vi "configuration UI.vi"() -> ()   [LabVIEW 2013, in "alarms module editor node.lvclass"]
uses:
  alarms module editor node.lvclass
  <vilib>/NI/Module Execution Interface/Engine Configuration/engine configuration.lvclass
  <vilib>/NI/Tag Bus Data Framework/Configuration Editor/Classes/Module editor node/module editor node.lvclass
  <vilib>/NI/Tag Bus Data Framework/Configuration Editor/Classes/Engine Parent/Engine Parent Editor Node.lvclass
  <vilib>/NI/Configuration Framework/serializable configuration/NISE_CEF_serializable configuration.lvclass
  module/configuration/alarms module configuration.lvclass
  <vilib>/NI/Tools/Keyed Array/KeyedArray.ctl
  <vilib>/NI/Tools/Keyed Array/Tools_KeyedArray.lvlib
  <vilib>/NI/AMC/Message.ctl
  <vilib>/NI/AMC/AMC.lvlib
  <vilib>/NI/AMC/Message Queue.ctl
  <vilib>/NI/Configuration Framework/Node/NISE_CEF_Node.lvclass
  <vilib>/NI/Configuration Framework/Node/NodeRef.ctl
  <vilib>/NI/Configuration Framework/Controls/EventCluster.ctl
  <vilib>/NI/Configuration Framework/NISE_CEF_TreeControl.lvlib
  <vilib>/NI/Configuration Framework/Node/UserEventRef.ctl
  <vilib>/NI/Configuration Framework/Node/StopEvent.ctl
  <vilib>/NI/Configuration Framework/Node/RefreshUIEvent.ctl
  <vilib>/NI/Configuration Framework/Node/CacheState.ctl
  <vilib>/NI/Configuration Framework/Node/NodeChangeEvent.ctl
panel:
  in  "node change":T1
  in  "cache state":T2
  in  "refresh UI":T3
  in  "stop event":T4
  in  "Tab Control":enum32{"Alarm Configuration", "Alarm Table"}(tab)
  in  "Alarms":i32(listbox)
  in  "Remove alarm":bool
  in  "Add alarm":bool
  in  "Full Alarms Table":i32(listbox)
  in  "user event":T5
  in  "main queue":T6
  in  "node ref":T7
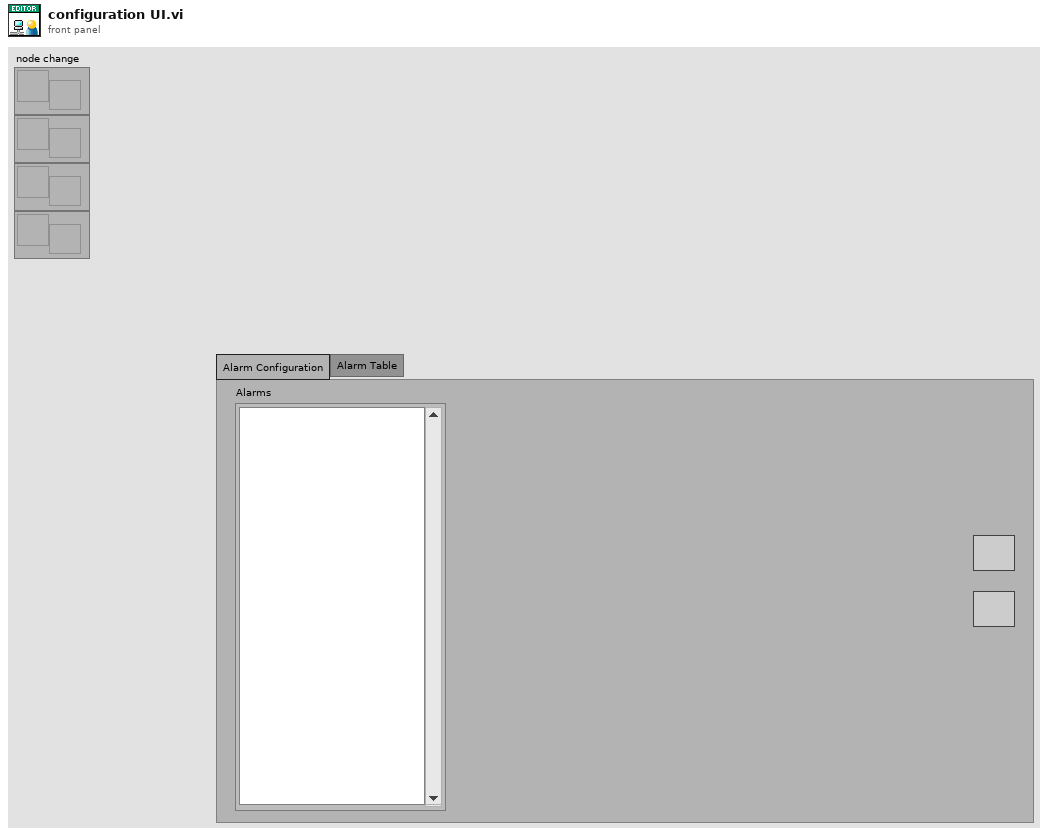
[diagram p1: front panel]
types:
  T1 = typedef "NISE_CEF_Node.lvclass/NodeChangeEvent.ctl" = refnum<user-event>
  T2 = typedef "NISE_CEF_Node.lvclass/CacheState.ctl" = refnum<user-event>
  T3 = typedef "NISE_CEF_Node.lvclass/RefreshUIEvent.ctl" = refnum<user-event>
  T4 = typedef "NISE_CEF_Node.lvclass/StopEvent.ctl" = refnum<user-event>
  T5 = typedef "NISE_CEF_Node.lvclass/UserEventRef.ctl" = refnum<user-event>
  T6 = typedef "AMC.lvlib/Message Queue.ctl" = refnum<queue>
  T7 = typedef "NISE_CEF_Node.lvclass/NodeRef.ctl" = refnum<data-value>
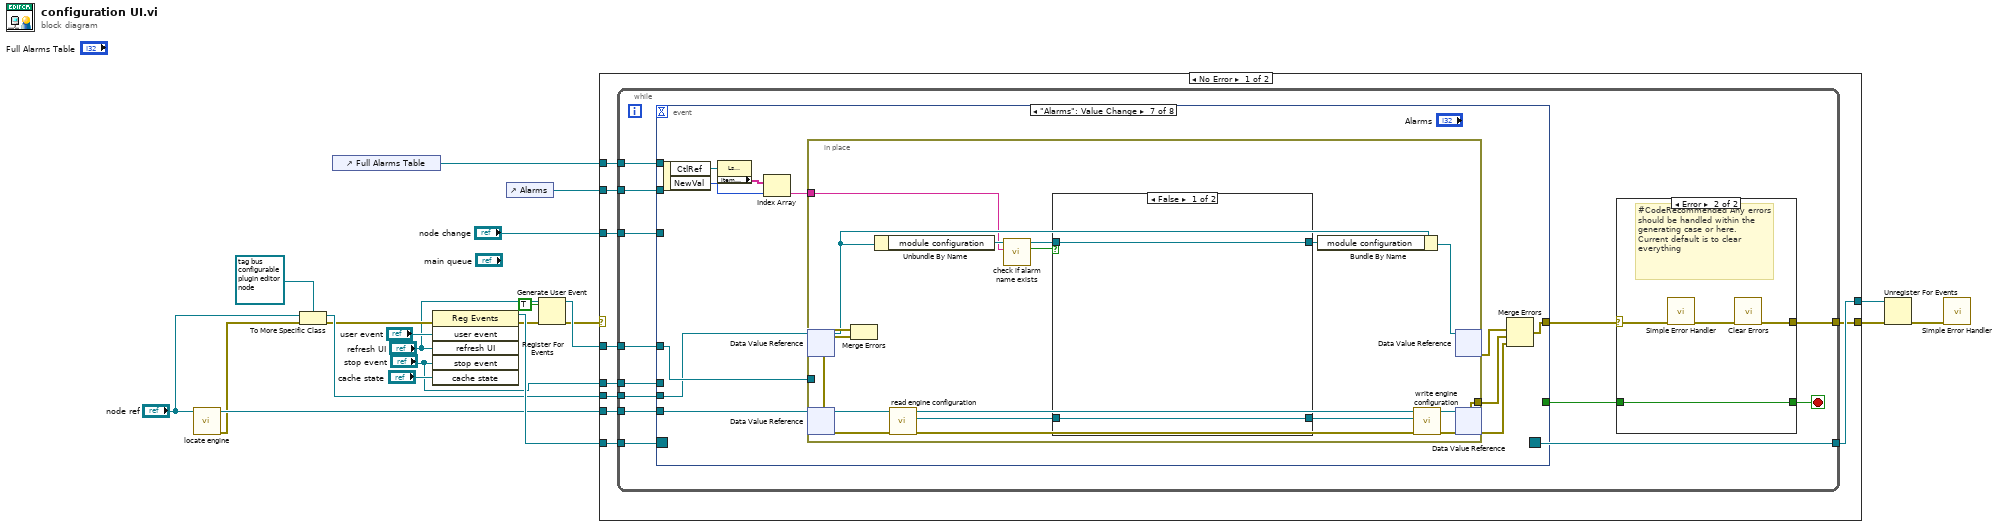
[diagram p0: block diagram]
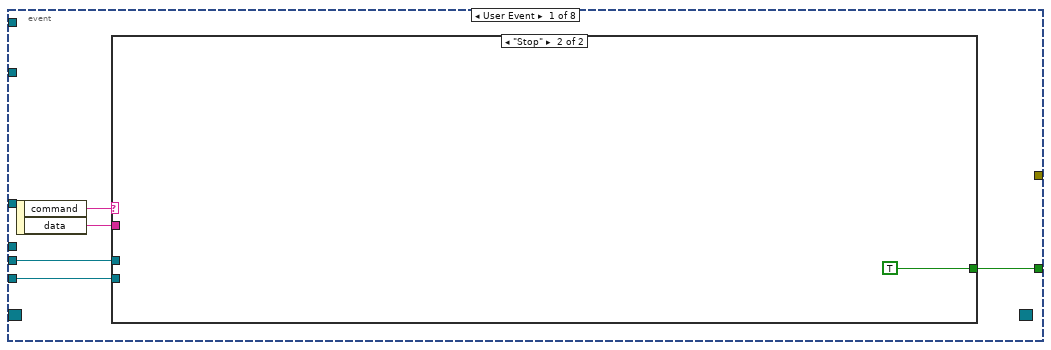
[diagram p3: hidden frame]
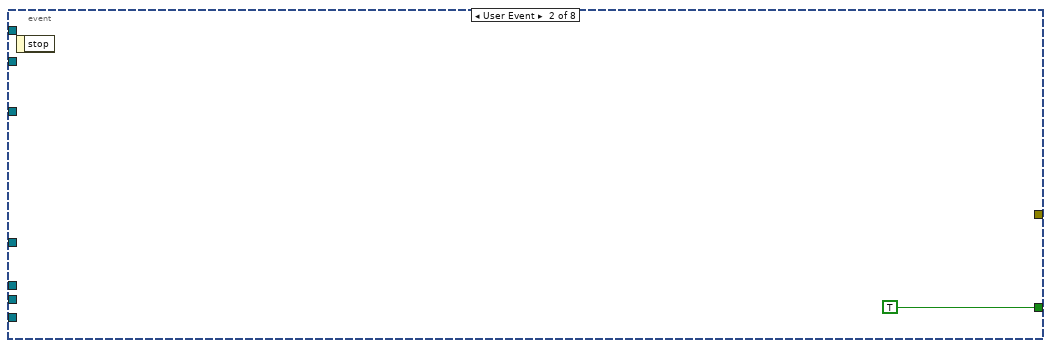
[diagram p5: hidden frame]
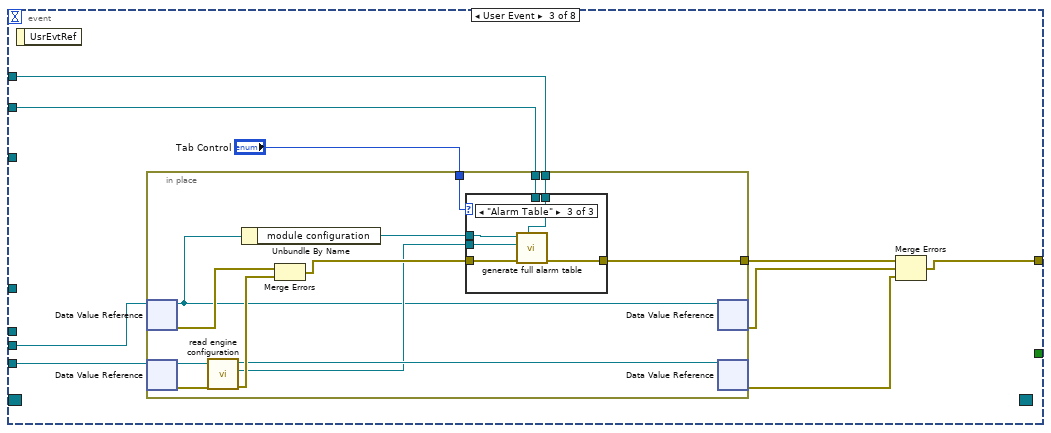
[diagram p6: hidden frame]
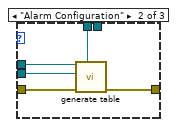
[diagram p8: hidden frame]
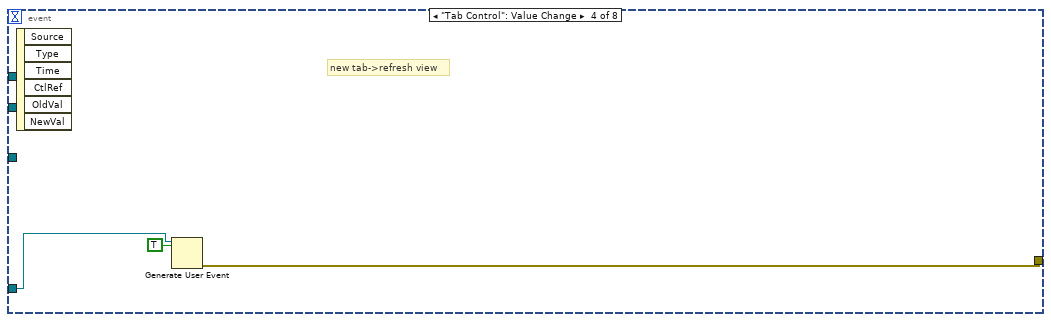
[diagram p9: hidden frame]
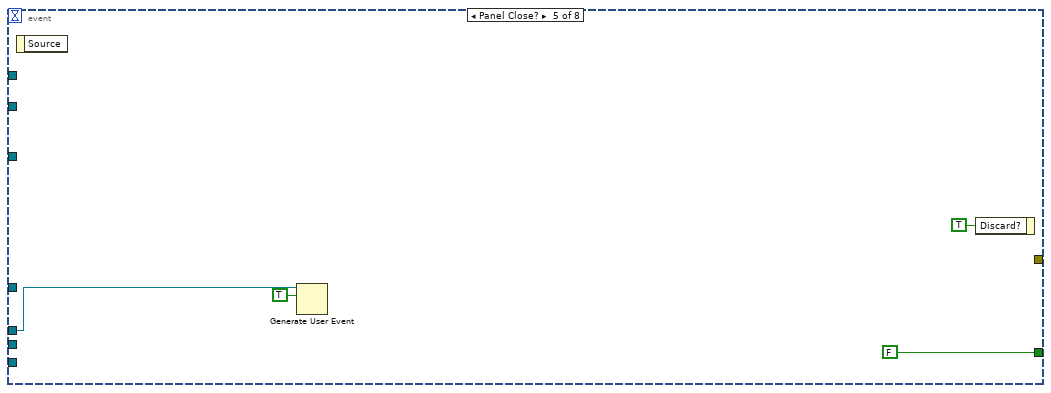
[diagram p10: hidden frame]
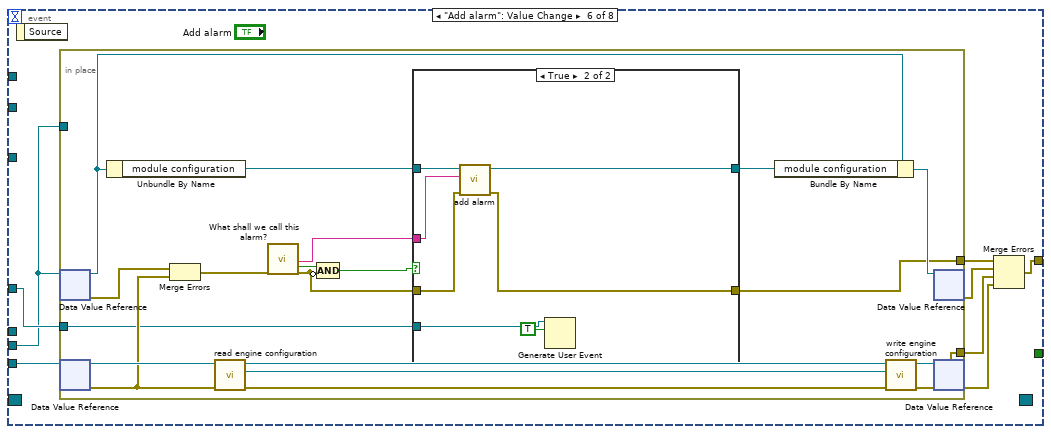
[diagram p11: hidden frame]
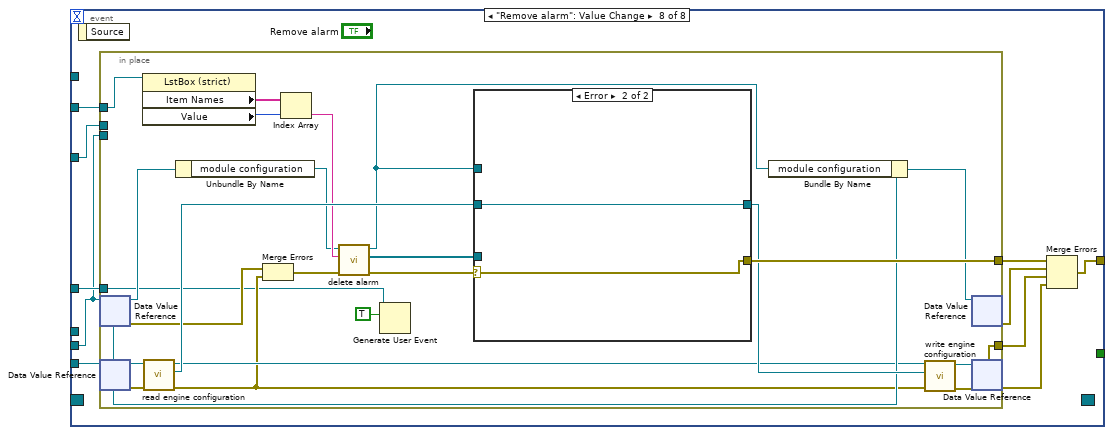
[diagram p14: hidden frame]
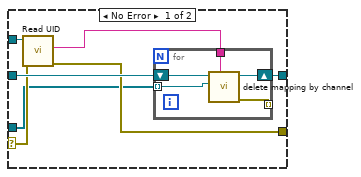
[diagram p15: hidden frame]
diagram:
  n1 = call <vilib>:"locate engine.vi"("component"="node ref") -> ("error out"=w10:errorcluster, "engine"=w16:refnum<data-value>)  [unwired: 9 in]
  n2 = To More Specific Class(target class=refnum<data-value> refnum ("data value reference"), reference="node ref", error in=w10) -> (specific class reference=w13:refnum<data-value>, error out=w12:errorcluster)
  n3 = control-ref of="Full Alarms Table"() -> (w1:refnum<vi>)
  n4 = register-events(error in=w12, "user event", "refresh UI", "stop event", "cache state") -> (reference out=w21:refnum<event-registration>, error out=w17:errorcluster)  [unwired: 1 in]
  n5 = control-ref of="Alarms"() -> (w2:refnum<vi>)
  n6 = Generate User Event(user event="refresh UI", event data cluster=TRUE ("event data"), error in=w17) -> (user event out=w9:T3, error out=w4:errorcluster)  [unwired: 1 in]
  n7 = case shown="No Error" w4 {
    selector: w4 -> [_ w211]
    tunnel: w21 -> [w31 w210]
    tunnel: [w30 w210] -> w20
    tunnel: [w29 w211] -> w19
    tunnel: w16 -> [w28 _]
    tunnel: w13 -> [w27 _]
    tunnel: w9 -> [w26 _]
    tunnel: "node change" -> [w25 _]
    tunnel: "stop event" -> [w24 _]
    tunnel: w2 -> [w23 _]
    tunnel: w1 -> [w22 _]
    frame No Error {
      n8 = while {
        tunnel: w31 -> [w44]
        tunnel: [w43] -> w30
        tunnel: w27 -> [w39]
        tunnel: w28 -> [w38]
        tunnel: w26 -> [w37]
        tunnel: w25 -> [w35]
        tunnel: [w40] -> w29
        tunnel: w24 -> [w34]
        tunnel: w23 -> [w33]
        tunnel: w22 -> [w32]
        stop <- w42 stop-if-true
        n9 = event shown="[6] \"Alarms\": Value Change" {
          selector: w44 -> [_ _ _ _ _ _ _ _]
          dyn-events: [_ _ _ _ _ _ _ _] -> w43
          timeout: _ -> [_ _ _ _ _ _ _ _]
          tunnel: [w55 TRUE _ _ FALSE _ _ _] -> w41
          tunnel: [_ _ w64 w91 _ w104 w143 w169] -> w36
          tunnel: w39 -> [w53 _ w66 _ _ w99 w138 w164]
          tunnel: w38 -> [w52 _ w65 _ _ w103 w142 w170]
          tunnel: w37 -> [_ _ _ w92 _ w105 w144 w171]
          tunnel: w35 -> [_ _ _ _ _ _ _ w165]
          tunnel: w34 -> [_ _ _ _ w95 _ _ _]
          tunnel: w33 -> [_ _ w59 _ _ _ _ w163]
          tunnel: w32 -> [_ _ w58 _ _ _ _ _]
          event User Event {
            n10 = event-data() -> ("command"=w54:string, "data"=w51:string)  [unwired: 1 in]
            n11 = case shown="\"Stop\"" w54 {
              tunnel: [_ TRUE] -> w55
              tunnel: w53 -> [_ _]
              tunnel: w52 -> [_ _]
              tunnel: w51 -> [_ _]
              frame Default {
              }
              frame "Stop" {
              }
            }
          }
          event User Event {
            n12 = event-data() -> ()  [unwired: 1 in, 1 out]
          }
          event User Event {
            n13 = event-data() -> ()  [unwired: 1 in, 1 out]
            n14 = in-place {
              in-place-border: [w79] -> w63
              in-place-border: "Tab Control" -> [w69]
              in-place-border: w59 -> [w68]
              in-place-border: w58 -> [w67]
              n15 = in-place-dvr #1(w66) -> (w71:refnum<class "alarms module editor node.lvclass">, w77:errorcluster)
              n16 = in-place-dvr #2(w65) -> (w74:refnum<class "Engine Parent Editor Node.lvclass">, w76:errorcluster)
              n17 = call <vilib>:"read engine configuration.vi"("error in"=w76, "Engine Parent Editor Node in"=w74) -> ("error out"=w75:errorcluster, "engine configuration"=w72:refnum<class "engine configuration.lvclass">, "Engine Parent Editor Node out"=w73:refnum<class "Engine Parent Editor Node.lvclass">)  [unwired: 7 in]
              n18 = Unbundle By Name(w71) -> ("module configuration"=w70:refnum<class "alarms module configuration.lvclass">)
              n19 = Merge Errors(w77, w75) -> (w78:errorcluster)
              n20 = case shown="\"Alarm Table\"" w69 {
                tunnel: [w80 w85 w89] -> w79
                tunnel: w78 -> [w80 w84 w90]
                tunnel: w72 -> [_ w83 w86]
                tunnel: w70 -> [_ w82 w87]
                tunnel: w68 -> [_ w81 _]
                tunnel: w67 -> [_ _ w88]
                frame Default {
                }
                frame "Alarm Configuration" {
                  n21 = call "generate table.vi"("Alarms list"=w81, "error in"=w84, "engine configuration"=w83, "tag bus configurable plugin module configuration"=w82) -> ("error out"=w85:errorcluster)  [unwired: 7 in]
                }
                frame "Alarm Table" {
                  n22 = call "generate full alarm table.vi"("Full Alarms Table"=w88, "error in"=w90, "engine configuration"=w86, "tag bus configurable plugin module configuration"=w87) -> ("error out"=w89:errorcluster)  [unwired: 7 in]
                }
              }
              n23 = in-place-dvr #1(w71) -> (w62:errorcluster)  [unwired: 1 out]
              n24 = in-place-dvr #2(w73) -> (w61:errorcluster)  [unwired: 1 out]
            }
            n25 = Merge Errors(w63, w62, w61) -> (w64:errorcluster)
          }
          event "Tab Control": Value Change {
            # "new tab->refresh view"
            n26 = event-data() -> ()  [unwired: 1 in, 6 out]
            n27 = Generate User Event(user event=w92, event data cluster=TRUE ("event data")) -> (error out=w91:errorcluster)  [unwired: 2 in, 1 out]
          }
          event Panel Close? {
            n28 = event-data() -> ()  [unwired: 1 in, 1 out]
            n29 = Generate User Event(user event=w95, event data cluster=TRUE ("event data")) -> ()  [unwired: 2 in, 2 out]
            n30 = event-data("Discard?"=TRUE) -> ()  [unwired: 1 in, 1 out]
          }
          event "Add alarm": Value Change {
            n31 = event-data() -> ()  [unwired: 1 in, 1 out]
            n32 = in-place {
              in-place-border: w105 -> [w106]
              in-place-border: [w121] -> w101
              in-place-border: w99 -> [_]
              in-place-border: [w109] -> w98
              n33 = in-place-dvr #3(w99) -> (w117:refnum<class "alarms module editor node.lvclass">, w118:errorcluster)
              n34 = in-place-dvr #4(w103) -> (w124:refnum<class "Engine Parent Editor Node.lvclass">, w123:errorcluster)
              n35 = Unbundle By Name(w117) -> ("module configuration"=w110:refnum<class "alarms module configuration.lvclass">)
              n36 = Merge Errors(w118, w123) -> (w115:errorcluster)
              n37 = call <vilib>:"read engine configuration.vi"("error in"=w123, "Engine Parent Editor Node in"=w124) -> ("error out"=w119:errorcluster, "engine configuration"=w107:refnum<class "engine configuration.lvclass">, "Engine Parent Editor Node out"=w120:refnum<class "Engine Parent Editor Node.lvclass">)  [unwired: 7 in]
              n38 = call "What shall we call this alarm?"("error in (no error)"=w115) -> ("Alarm Name"=w108:string, "OK"=w114:bool, "error out"=w113:errorcluster)  [unwired: 16 in]
              n39 = Compound Arithmetic op=AND(w114, invert w113) -> (w112:bool)
              n40 = case shown="True" w112 {
                tunnel: w113 -> [w125 w132]
                tunnel: [w126 w131] -> w111
                tunnel: w110 -> [w126 w133]
                tunnel: [w125 w129] -> w109
                tunnel: w108 -> [_ w130]
                tunnel: w106 -> [_ w128]
                frame False {
                }
                frame True {
                  n41 = call "add alarm.vi"("error in"=w132, "alarm name"=w130, "alarms module configuration in"=w133) -> ("error out"=w129:errorcluster, "alarms module configuration out"=w131:refnum<class "alarms module configuration.lvclass">)  [unwired: 6 in, 1 out]
                  n42 = Generate User Event(user event=w128, event data cluster=TRUE ("event data")) -> ()  [unwired: 2 in, 2 out]
                }
              }
              n43 = Bundle By Name(cluster=w117, "module configuration"=w111) -> (w116:refnum<class "alarms module editor node.lvclass">)
              n44 = call <vilib>:"write engine configuration.vi"("error in"=w119, "engine configuration"=w107, "Engine Parent Editor Node in"=w120) -> ("error out"=w121:errorcluster, "Engine Parent Editor Node out"=w122:refnum<class "Engine Parent Editor Node.lvclass">)  [unwired: 7 in]
              n45 = in-place-dvr #3(w116) -> (w100:errorcluster)  [unwired: 1 out]
              n46 = in-place-dvr #4(w122) -> (w102:errorcluster)  [unwired: 1 out]
            }
            n47 = Merge Errors(w98, w100, w101, w102) -> (w104:errorcluster)
          }
          event "Alarms": Value Change {
            n48 = event-data() -> ("CtlRef"=w136:refnum<vi>, "NewVal"=w135:i32)  [unwired: 1 in]
            n49 = property class="LstBox (strict)"(reference=w136) -> ("Item Names"=w137:string[])  [unwired: 1 in, 2 out]
            n50 = Index Array(array=w137, index=w135) -> (element=w134:string)
            n51 = in-place {
              in-place-border: w144 -> [_]
              in-place-border: [w157] -> w140
              in-place-border: w134 -> [w150]
              n52 = in-place-dvr #5(w138) -> (w153:refnum<class "alarms module editor node.lvclass">, w154:errorcluster)
              n53 = in-place-dvr #6(w142) -> (w160:refnum<class "Engine Parent Editor Node.lvclass">, w159:errorcluster)
              n54 = Merge Errors(w154, w159) -> ()  [unwired: 1 out]
              n55 = Unbundle By Name(w153) -> ("module configuration"=w151:refnum<class "alarms module configuration.lvclass">)
              n56 = call <vilib>:"read engine configuration.vi"("error in"=w159, "Engine Parent Editor Node in"=w160) -> ("error out"=w155:errorcluster, "engine configuration"=w146:refnum<class "engine configuration.lvclass">, "Engine Parent Editor Node out"=w156:refnum<class "Engine Parent Editor Node.lvclass">)  [unwired: 7 in]
              n57 = call "check if alarm name exists.vi"("name to locate"=w150, "alarms module configuration in"=w151) -> ("found?"=w149:bool, "alarms module configuration out"=w148:refnum<class "alarms module configuration.lvclass">)  [unwired: 6 in, 2 out]
              n58 = case shown="False" w149 {
                tunnel: w148 -> [w162 _]
                tunnel: [w162 _] -> w147
                tunnel: w146 -> [w161 _]
                tunnel: [w161 _] -> w145
                frame False {
                }
                frame True {
                }
              }
              n59 = Bundle By Name(cluster=w153, "module configuration"=w147) -> (w152:refnum<class "alarms module editor node.lvclass">)
              n60 = call <vilib>:"write engine configuration.vi"("error in"=w155, "engine configuration"=w145, "Engine Parent Editor Node in"=w156) -> ("error out"=w157:errorcluster, "Engine Parent Editor Node out"=w158:refnum<class "Engine Parent Editor Node.lvclass">)  [unwired: 7 in]
              n61 = in-place-dvr #5(w152) -> (w139:errorcluster)  [unwired: 1 out]
              n62 = in-place-dvr #6(w158) -> (w141:errorcluster)  [unwired: 1 out]
            }
            n63 = Merge Errors(w139, w140, w141) -> (w143:errorcluster)  [unwired: 1 in]
          }
          event "Remove alarm": Value Change {
            n64 = event-data() -> ()  [unwired: 1 in, 1 out]
            n65 = in-place {
              in-place-border: [w195] -> w172
              in-place-border: w171 -> [w175]
              in-place-border: [w193] -> w166
              in-place-border: w165 -> [_]
              in-place-border: w164 -> [_]
              in-place-border: w163 -> [w183]
              n66 = in-place-dvr #7(w164) -> (w188:refnum<class "alarms module editor node.lvclass">, w184:errorcluster)
              n67 = in-place-dvr #8(w170) -> (w190:refnum<class "Engine Parent Editor Node.lvclass">, w189:errorcluster)
              n68 = property class="LstBox (strict)"(reference=w183) -> ("Item Names"=w181:string[], "Value"=w182:i32)  [unwired: 1 in, 2 out]
              n69 = call <vilib>:"read engine configuration.vi"("error in"=w189, "Engine Parent Editor Node in"=w190) -> ("error out"=w185:errorcluster, "engine configuration"=w187:refnum<class "engine configuration.lvclass">, "Engine Parent Editor Node out"=w186:refnum<class "Engine Parent Editor Node.lvclass">)  [unwired: 7 in]
              n70 = Unbundle By Name(w188) -> ("module configuration"=w178:refnum<class "alarms module configuration.lvclass">)
              n71 = Merge Errors(w184, w185) -> (w180:errorcluster)
              n72 = Index Array(array=w181, index=w182) -> (element=w179:string)
              n73 = call "delete alarm.vi"("error in"=w180, "alarm name"=w179, "alarms module configuration in"=w178) -> ("error out"=w177:errorcluster, "deleted channels"=w174:refnum<class "TBM channel.lvclass">[], "alarms module configuration out"=w173:refnum<class "alarms module configuration.lvclass">)  [unwired: 6 in]
              n74 = Generate User Event(user event=w175, event data cluster=TRUE ("event data")) -> ()  [unwired: 2 in, 2 out]
              n75 = case shown="Error" w177 {
                selector: w177 -> [w198 w208]
                tunnel: [w197 w208] -> w195
                tunnel: w173 -> [w200 _]
                tunnel: w187 -> [w202 w209]
                tunnel: [w201 w209] -> w191
                tunnel: w174 -> [w196 _]
                frame No Error {
                  n76 = call <vilib>:"Read UID.vi"("error in"=w198, "configuration in"=w200) -> ("error out"=w197:errorcluster, "instance id"=w199:string)  [unwired: 7 in, 1 out]
                  n77 = for {
                    tunnel: w199 -> [w205]
                    shift-right: [w206] -> w201
                    shift-left: w202 -> [w207]
                    tunnel: [w204] -> _ mode=indexing
                    tunnel: w196 -> [w203] mode=indexing
                    n78 = call <vilib>:"delete mapping by channel.vi"("owner ID"=w205, "channel"=w203, "engine configuration in"=w207) -> ("error out"=w204:errorcluster, "engine configuration out"=w206:refnum<class "engine configuration.lvclass">)  [unwired: 7 in]
                  }
                }
                frame Error {
                }
              }
              n79 = Bundle By Name(cluster=w188, "module configuration"=w173) -> (w192:refnum<class "alarms module editor node.lvclass">)
              n80 = call <vilib>:"write engine configuration.vi"("error in"=w185, "engine configuration"=w191, "Engine Parent Editor Node in"=w186) -> ("error out"=w193:errorcluster, "Engine Parent Editor Node out"=w194:refnum<class "Engine Parent Editor Node.lvclass">)  [unwired: 7 in]
              n81 = in-place-dvr #7(w192) -> (w167:errorcluster)  [unwired: 1 out]
              n82 = in-place-dvr #8(w194) -> (w168:errorcluster)  [unwired: 1 out]
            }
            n83 = Merge Errors(w172, w167, w166, w168) -> (w169:errorcluster)
          }
        }
        n84 = case shown="Error" w36 {
          selector: w36 -> [w45 w49]
          tunnel: [w46 w50] -> w42
          tunnel: w41 -> [w46 w50]
          tunnel: [w45 w47] -> w40
          frame No Error {
          }
          frame Error {
            # "#CodeRecommended Any errors should be handled within the generating case or here. Current default is to clear everything"
            n85 = call <vilib>:"Simple Error Handler.vi"("error in (no error)"=w49) -> ("error out"=w48:errorcluster)  [unwired: 4 in, 4 out]
            n86 = call <vilib>:"Clear Errors.vi"("error in (no error)"=w48) -> ("error out"=w47:errorcluster)  [unwired: 6 in]
          }
        }
      }
    }
    frame Error {
    }
  }
  n87 = Unregister For Events(event registration refnum=w20, error in=w19) -> (error out=w15:errorcluster)
  n88 = call <vilib>:"Simple Error Handler.vi"("error in (no error)"=w15) -> ()  [unwired: 4 in, 5 out]
